vi "Periodic Tasks.vi"(8 "error in":errorcluster) -> ()   [LabVIEW 2017]
doc: "This VI runs in parallel to other tasks. It can contain as many user-defined periodic loops as you need. These can carry out PID or other sorts of timed response."
uses:
  <vilib>/Rock Robotics/WPI/Solenoid/WPI_SolenoidValue.ctl
  <vilib>/Rock Robotics/WPI/ThirdParty/Phoenix-LabVIEW/Motor Controller/Controls/CTRE_Phoenix_MotorControl_ControlMode.ctl
  <vilib>/Rock Robotics/WPI/DriverStation/WPI_DriverStationRobotMode2.ctl
  LabVIEW_is_Under_Control.lib/Util/Toggle/Change Detect.vi
  LabVIEW_is_Under_Control.lib/Util/Toggle/Change Detect Boolean.vi
  Robot Global Data.vi
  <vilib>/Rock Robotics/WPI/Solenoid/WPI_SolenoidSetEnum.vi
panel:
  in  "Exchange":dbl
  in  "ScoringHigh":dbl
  in  "Scoring Low":dbl
  in  "Reset":bool
  in  "Gains Elevador":T1={"proportional gain (Kc)"=1.0, "integral time (Ti, min)"=0.01, "derivative time (Td, min)"=0.0} {"derivative time (Td, min)" format="%.3f"; "integral time (Ti, min)" format="%.3f"; "proportional gain (Kc)" format="%.3f"}
  in  "Range Elevador":cluster{"output high":dbl, "output low":dbl}={"output high"=0.6, "output low"=-0.6} {"output low" format="%.2f"; "output high" format="%.2f"}
  in  "Enable squared":bool
  in  "Score":dbl=-0.3
  in  "Segurando":dbl=0.3
  in  "Expelir":dbl=-0.3
  in  "Coletar":dbl=0.9
  # "Intake"
  # "Drivetrain"
  # "Elevador"
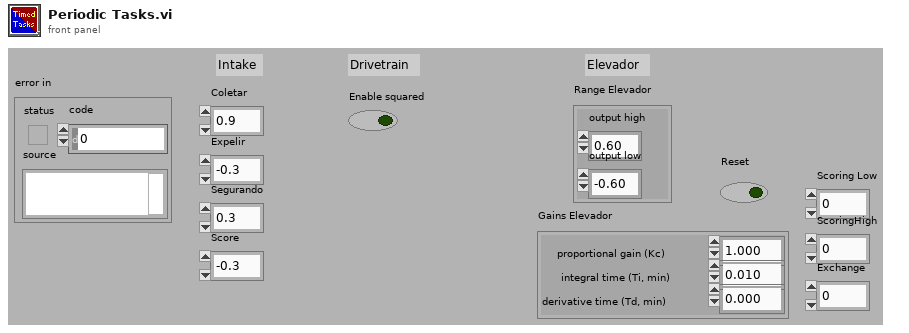
[diagram p1: front panel]
types:
  T1 = cluster{"proportional gain (Kc)":dbl, "integral time (Ti, min)":dbl, "derivative time (Td, min)":dbl}
  T2 = typedef "Máquina de estado do elevador.ctl" = enum16{"Resting", "Scoring Low", "Scoring Higher", "Exchange"}
  T3 = enum16{"Repouso", "Coletando", "Segurando", "Score"}
  T4 = typedef "WPI_SwitchDevRef.ctl" = cluster{"DevStatus":errorcluster, "DIO Channel":T5, "CntIndex":T6, "Normally Closed":bool}
  T5 = typedef "FPGA_DIOChannel.ctl" = enum8{"DIO 0", "DIO 1", "DIO 2", "DIO 3", "DIO 4", "DIO 5", "DIO 6", "DIO 7", "DIO 8", "DIO 9", "DIO MXP 0", "DIO MXP 1", "DIO MXP 2", "DIO MXP 3", "DIO MXP 4", "DIO MXP 5", "DIO MXP 6", "DIO MXP 7", "DIO MXP 8", "DIO MXP 9", "DIO MXP 10", "DIO MXP 11", "DIO MXP 12", "DIO MXP 13", "DIO MXP 14", "DIO MXP 15", "SPI Port CS1", "SPI Port CS2", "SPI Port CS3", "SPI Port MISO", "SPI Port MOSI", "Invalid"}
  T6 = typedef "FPGA_CounterCtrSystemIndex.ctl" = enum8{"Ctr 0", "Ctr 1", "Ctr 2", "Ctr 3", "Ctr 4", "Ctr 5", "Ctr 6", "Ctr 7", "Invalid"}
  T7 = typedef "WPI_EncoderDevRef.ctl" = cluster{"DevStatus":errorcluster, "EncoderIndex":T8, "CounterIndex":T6, "DistancePerCount":dbl, "Decoding Type":T9}
  T8 = typedef "FPGA_EncoderIdx.ctl" = enum8{"Enc 0", "Enc 1", "Enc 2", "Enc 3", "Enc 4", "Enc 5", "Enc 6", "Enc 7", "Invalid"}
  T9 = typedef "WPI_EncoderType.ctl" = enum16{"1x", "2x", "4x"}
  T10 = typedef "WPI_SolenoidDevRef.ctl" = cluster{"DevStatus":errorcluster, "Pneumatics Control Module":u8, "Forward Solenoid Channel":T11, "Reverse Solenoid Channel":T11}
  T11 = typedef "WPI_SolenoidChannel.ctl" = enum8{"Solenoid 0", "Solenoid 1", "Solenoid 2", "Solenoid 3", "Solenoid 4", "Solenoid 5", "Solenoid 6", "Solenoid 7", "Invalid"}
  T12 = typedef "WPI_MotorControlDeviceRef.ctl" = cluster{"DeviceStatus":errorcluster, "Type":T13, "PWM":cluster{"PWM Channel":T14, "DeadBand":T15}, "CAN":cluster{"Device Number":u8, "SetOutput VI Ref":variant, "GetOutput VI Ref":variant, "Enable VI Ref":variant, "Disable VI Ref":variant, "Data":variant}, "Invert":bool, "DIO PWM":cluster{"PWM \"Enable\" Channel":T14, "DIOChannel":T5, "PWM Rate":dbl}}
  T13 = typedef "WPI_MotorControlType.ctl" = enum16{"PWM", "CAN", "DIO PWM"}
  T14 = typedef "FPGA_DIOPWMChannel.ctl" = enum8{"PWM 0", "PWM 1", "PWM 2", "PWM 3", "PWM 4", "PWM 5", "PWM 6", "PWM 7", "PWM 8", "PWM 9", "PWM MXP 0", "PWM MXP 1", "PWM MXP 2", "PWM MXP 3", "PWM MXP 4", "PWM MXP 5", "PWM MXP 6", "PWM MXP 7", "PWM MXP 8", "PWM MXP 9", "Invalid"}
  T15 = typedef "WPI_PWMDeadband.ctl" = cluster{"Name":string, "maxPositivePwm":i32, "minPositivePwm":i32, "centerPwm":i32, "maxNegativePwm":i32, "minNegativePwm":i32, "angularRange":u16}
  T16 = typedef "WPI_SolenoidValue.ctl" = enum16{"Off", "On", "Forward", "Reverse"}
  T17 = typedef "WPI_DriverStationRobotMode2.ctl" = enum16{"Autonomous Disabled", "Autonomous Enabled", "Teleop Disabled", "Teleop Enabled", "Disconnected", "Finish", "Test Disabled", "Test Enabled", "Emergency Stopped"}
  T18 = typedef "CTRE_Phoenix_MotorControl_ControlMode.ctl" = u16
  T19 = typedef "Axes Cluster.ctl" = cluster{"Axes[0]":dbl, "Axes[1]":dbl, "Axes[2]":dbl, "Axes[3]":dbl, "Axes[4]":dbl, "Axes[5]":dbl, "Axes[6]":dbl, "Axes[7]":dbl, "Axes[8]":dbl}
  T20 = typedef "Button Cluster.ctl" = cluster{"Buttons[0]":bool, "Buttons[1]":bool, "Buttons[2]":bool, "Buttons[3]":bool, "Buttons[4]":bool, "Buttons[5]":bool, "Buttons[6]":bool, "Buttons[7]":bool, "Buttons[8]":bool, "Buttons[9]":bool}
  T21 = typedef "D-Pad.ctl" = cluster{"Top":bool, "Bottom":bool, "None":bool, "Right":bool, "Left":bool}
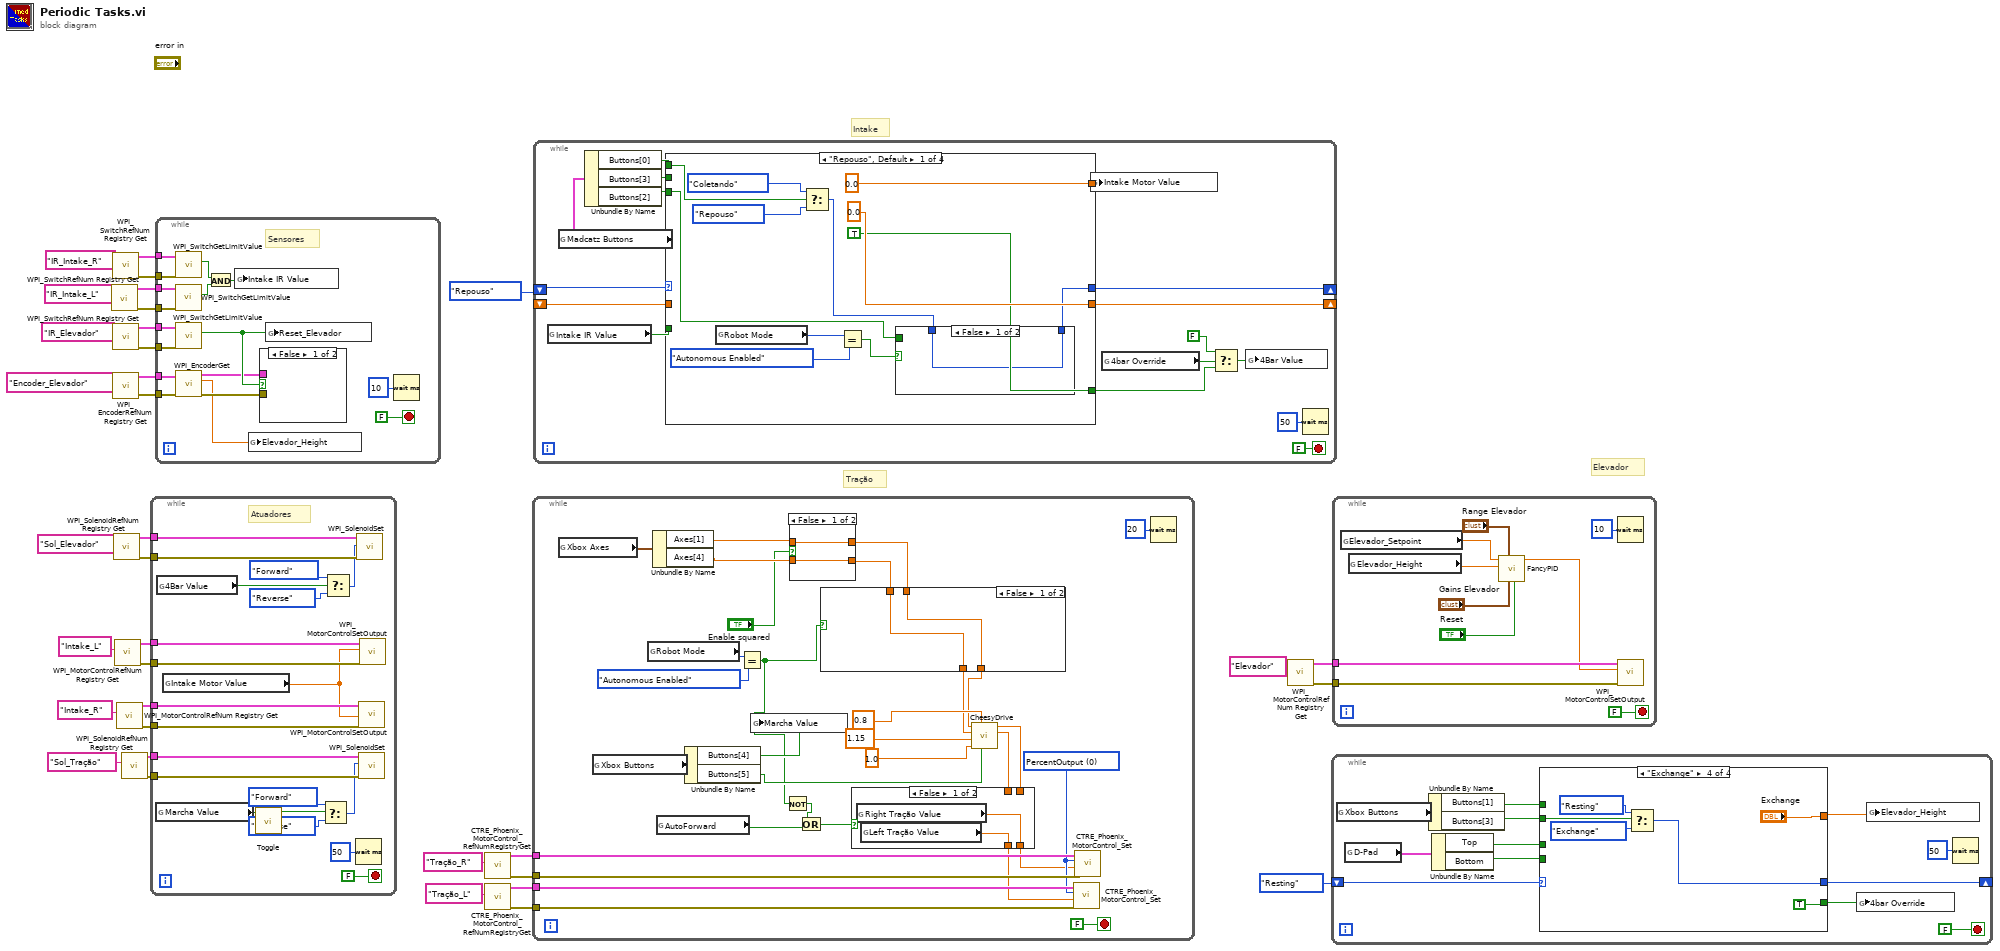
[diagram p0: block diagram]
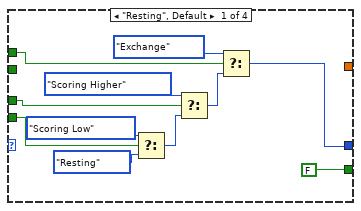
[diagram p2: hidden frame]
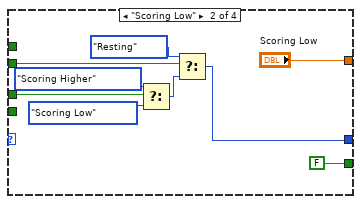
[diagram p3: hidden frame]
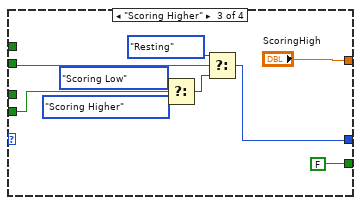
[diagram p4: hidden frame]
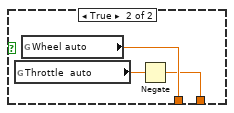
[diagram p6: hidden frame]
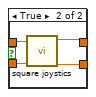
[diagram p7: hidden frame]
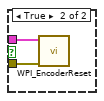
[diagram p8: hidden frame]
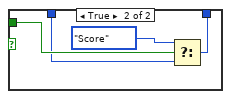
[diagram p9: hidden frame]
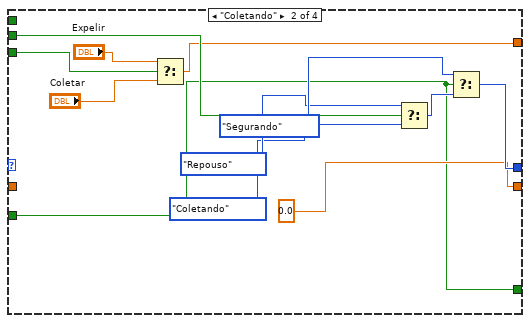
[diagram p10: hidden frame]
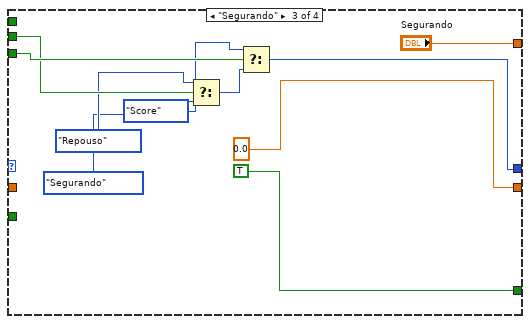
[diagram p11: hidden frame]
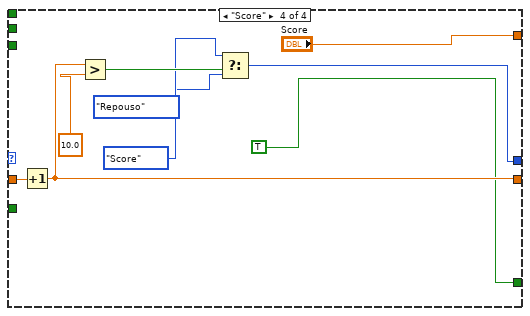
[diagram p12: hidden frame]
diagram:
  # "Elevador"
  # "Tração"
  # "Intake"
  n1 = call <vilib>:"WPI_SwitchRefNum Registry Get.vi"("refnum name"="IR_Intake_L") -> ("error out"=w32:errorcluster, "SwitchDevRef"=w31:T4)  [unwired: 9 in]
  n2 = call <vilib>:"WPI_SwitchRefNum Registry Get.vi"("refnum name"="IR_Intake_R") -> ("error out"=w30:errorcluster, "SwitchDevRef"=w29:T4)  [unwired: 9 in]
  n3 = call <vilib>:"WPI_SwitchRefNum Registry Get.vi"("refnum name"="IR_Elevador") -> ("error out"=w9:errorcluster, "SwitchDevRef"=w10:T4)  [unwired: 9 in]
  n4 = call <vilib>:"WPI_EncoderRefNum Registry Get.vi"("refnum name"="Encoder_Elevador") -> ("error out"=w5:errorcluster, "EncoderDevRef"=w6:T7)  [unwired: 9 in]
  n5 = call <vilib>:"WPI_SolenoidRefNum Registry Get.vi"("refnum name"="Sol_Elevador") -> ("error out"=w27:errorcluster, "SolenoidDevRef"=w26:T10)  [unwired: 9 in]
  n6 = call <vilib>:"WPI_MotorControlRefNum Registry Get.vi"("refnum name"="Intake_L") -> ("error out"=w25:errorcluster, "MotorControlDevRef"=w24:T12)  [unwired: 9 in]
  n7 = call <vilib>:"WPI_MotorControlRefNum Registry Get.vi"("refnum name"="Intake_R") -> ("error out"=w20:errorcluster, "MotorControlDevRef"=w21:T12)  [unwired: 9 in]
  n8 = call <vilib>:"WPI_SolenoidRefNum Registry Get.vi"("refnum name"="Sol_Tração") -> ("error out"=w17:errorcluster, "SolenoidDevRef"=w18:T10)  [unwired: 9 in]
  n9 = while {
    tunnel: w27 -> [w55]
    tunnel: w26 -> [w54]
    tunnel: w25 -> [w49]
    tunnel: w24 -> [w48]
    tunnel: w21 -> [w47]
    tunnel: w20 -> [w46]
    tunnel: w18 -> [w40]
    tunnel: w17 -> [w39]
    stop <- FALSE stop-if-true
    # "Atuadores"
    n10 = global read "Robot Global Data.vi" "Marcha Value"() -> (w37:bool)
    n11 = global read "Robot Global Data.vi" "4Bar Value"() -> (w50:bool)
    n12 = global read "Robot Global Data.vi" "Intake Motor Value"() -> (w45:dbl)
    n13 = call "Toggle.vi"("In"=w37) -> ("Toggled"=w36:bool)  [unwired: 10 in]
    n14 = Select(t=WPI_SolenoidValue."Forward" ("Value"), s=w36, f=WPI_SolenoidValue."Reverse" ("Value")) -> (s? t:f=w38:T16)
    n15 = Select(t=WPI_SolenoidValue."Forward" ("Value"), s=w50, f=WPI_SolenoidValue."Reverse" ("Value")) -> (s? t:f=w53:T16)
    n16 = Wait (ms)(milliseconds to wait=u32 50) -> ()  [unwired: 1 out]
    n17 = call-poly <vilib>:"WPI_SolenoidSet.vi"("error in (no error)"=w55, "Value"=w53, "SolenoidDevRef"=w54) -> ()  [unwired: 7 in, 2 out]
    n18 = call <vilib>:"WPI_MotorControlSetOutput.vi"("error in (no error)"=w46, "Output"=w45, "MotorControlDevRef"=w47) -> ()  [unwired: 6 in, 3 out]
    n19 = call-poly <vilib>:"WPI_SolenoidSet.vi"("error in (no error)"=w39, "Value"=w38, "SolenoidDevRef"=w40) -> ()  [unwired: 7 in, 2 out]
    n20 = call <vilib>:"WPI_MotorControlSetOutput.vi"("error in (no error)"=w49, "Output"=w45, "MotorControlDevRef"=w48) -> ()  [unwired: 6 in, 3 out]
  }
  n21 = while {
    tunnel: w32 -> [w67]
    tunnel: w31 -> [w66]
    tunnel: w30 -> [w65]
    tunnel: w29 -> [w64]
    tunnel: w9 -> [w62]
    tunnel: w10 -> [w63]
    tunnel: w6 -> [w61]
    tunnel: w5 -> [w60]
    stop <- FALSE stop-if-true
    # "Sensores"
    n22 = call <vilib>:"WPI_SwitchGetLimitValue.vi"("error in (no error)"=w67, "SwitchDevRef"=w66) -> ("Switch Pressed"=w72:bool)  [unwired: 7 in, 2 out]
    n23 = call <vilib>:"WPI_SwitchGetLimitValue.vi"("error in (no error)"=w65, "SwitchDevRef"=w64) -> ("Switch Pressed"=w71:bool)  [unwired: 7 in, 2 out]
    n24 = call <vilib>:"WPI_SwitchGetLimitValue.vi"("error in (no error)"=w62, "SwitchDevRef"=w63) -> ("Switch Pressed"=w59:bool)  [unwired: 7 in, 2 out]
    n25 = call <vilib>:"WPI_EncoderGet.vi"("error in (no error)"=w60, "EncoderDevRef"=w61) -> ("error out"=w57:errorcluster, "Distance"=w56:dbl, "EncoderDevRef"=w58:T7)  [unwired: 4 in, 3 out]
    n26 = And(x=w71, y=w72) -> (x .and. y?=w68:bool)
    n27 = global write "Robot Global Data.vi" "Intake IR Value"(w68) -> ()
    n28 = global write "Robot Global Data.vi" "Elevador_Height"(w56) -> ()
    n29 = case shown="False" w59 {
      tunnel: w58 -> [_ w74]
      tunnel: w57 -> [_ w73]
      frame False {
      }
      frame True {
        n30 = call <vilib>:"WPI_EncoderReset.vi"("error in (no error)"=w73, "EncoderDevRef"=w74) -> ()  [unwired: 8 in, 2 out]
      }
    }
    n31 = global write "Robot Global Data.vi" "Reset_Elevador"(w59) -> ()
    n32 = Wait (ms)(milliseconds to wait=u32 10) -> ()  [unwired: 1 out]
  }
  n33 = call <vilib>:"CTRE_Phoenix_MotorControl_RefNumRegistryGet.vi"("refnum name"="Tração_R") -> ("error out"=w12:errorcluster, "PhoenixMotorControlDevRef"=w14:T12)  [unwired: 9 in]
  n34 = call <vilib>:"CTRE_Phoenix_MotorControl_RefNumRegistryGet.vi"("refnum name"="Tração_L") -> ("error out"=w11:errorcluster, "PhoenixMotorControlDevRef"=w13:T12)  [unwired: 9 in]
  n35 = while {
    tunnel: w14 -> [w96]
    tunnel: w13 -> [w95]
    tunnel: w12 -> [w94]
    tunnel: w11 -> [w93]
    stop <- FALSE stop-if-true
    w92 = T18 0 items=["PercentOutput"=0, "Position"=1, "Velocity"=2, "Current"=3, "Follower"=5, "MotionProfile"=6, "MotionMagic"=7, "MotionMagicArc"=8, "MotionProfileArc"=10, "Disabled"=15] ("Control Mode")
    n36 = global read "Robot Global Data.vi" "Xbox Axes"() -> (w105:T19)
    n37 = global read "Robot Global Data.vi" "Xbox Buttons"() -> (w103:T20)
    n38 = global read "Robot Global Data.vi" "Robot Mode"() -> (w88:T17)
    n39 = Unbundle By Name(w105) -> ("Axes[1]"=w90:dbl, "Axes[4]"=w91:dbl)
    n40 = global read "Robot Global Data.vi" "AutoForward"() -> (w76:bool)
    n41 = Unbundle By Name(w103) -> ("Buttons[4]"=w101:bool, "Buttons[5]"=w102:bool)
    n42 = Equal?(x=w88, y=WPI_DriverStationRobotMode2."Autonomous Enabled") -> (x = y?=w75:bool)
    n43 = global write "Robot Global Data.vi" "Marcha Value"(w101) -> ()
    n44 = Not(x=w75) -> (.not. x?=w78:bool)
    n45 = case shown="False" "Enable squared" {
      tunnel: w91 -> [w116 w120]
      tunnel: [w116 w119] -> w85
      tunnel: w90 -> [w115 w118]
      tunnel: [w115 w117] -> w86
      frame False {
      }
      frame True {
        n46 = call "square joystics.vi"("right joy"=w120, "left joy"=w118) -> ("Right Out"=w119:dbl, "Left Out"=w117:dbl)  [unwired: 8 in]
      }
    }
    n47 = Or(x=w78, y=w76) -> (x .or. y?=w77:bool)
    n48 = case shown="False" w75 {
      tunnel: [w110 w114] -> w79
      tunnel: [w111 w112] -> w80
      tunnel: w86 -> [w111 _]
      tunnel: w85 -> [w110 _]
      frame False {
      }
      frame True {
        n49 = global read "Robot Global Data.vi" "Throttle  auto"() -> (w113:dbl)
        n50 = global read "Robot Global Data.vi" "Wheel auto"() -> (w114:dbl)
        n51 = Negate(x=w113) -> (-x=w112:dbl)
      }
    }
    n52 = call "CheesyDrive.vi"("Quickturn"=w102, "WheelNonLinearity"=0.8, "negInertiaScalar"=1.0, "Sensitivty"=1.15, "Wheel"=w79, "Throttle"=w80) -> ("Right PWM"=w81:dbl, "Left PWM"=w83:dbl)  [unwired: 4 in]
    n53 = case shown="False" w77 {
      tunnel: [w106 w108] -> w84
      tunnel: w83 -> [_ w108]
      tunnel: [w107 w109] -> w82
      tunnel: w81 -> [_ w109]
      frame False {
        n54 = global read "Robot Global Data.vi" "Right Tração Value"() -> (w106:dbl)
        n55 = global read "Robot Global Data.vi" "Left Tração Value"() -> (w107:dbl)
      }
      frame True {
      }
    }
    n56 = call <vilib>:"CTRE_Phoenix_MotorControl_Set.vi"("error in (no error)"=w93, "Output"=w82, "Control Mode"=w92, "PhoenixMotorControlDevRef"=w95) -> ()  [unwired: 6 in, 2 out]
    n57 = call <vilib>:"CTRE_Phoenix_MotorControl_Set.vi"("error in (no error)"=w94, "Output"=w84, "Control Mode"=w92, "PhoenixMotorControlDevRef"=w96) -> ()  [unwired: 6 in, 2 out]
    n58 = Wait (ms)(milliseconds to wait=u32 20) -> ()  [unwired: 1 out]
  }
  n59 = while {
    shift-right: [w132] -> _
    shift-left: T3."Repouso" -> [w136]
    shift-right: [w129] -> _
    shift-left: _ -> [w130]
    stop <- FALSE stop-if-true
    n60 = global read "Robot Global Data.vi" "Intake IR Value"() -> (w131:bool)
    n61 = global read "Robot Global Data.vi" "Madcatz Buttons"() -> (w133:T20)
    n62 = Unbundle By Name(w133) -> ("Buttons[0]"=w125:bool, "Buttons[3]"=w127:bool, "Buttons[2]"=w126:bool)
    n63 = case shown="\"Repouso\", Default" w136 {
      tunnel: w125 -> [w148 _ _ _]
      tunnel: [w138 w161 w169 w178] -> w132
      tunnel: w127 -> [_ w164 w173 _]
      tunnel: w131 -> [_ w155 _ _]
      tunnel: w126 -> [w137 w154 w175 _]
      tunnel: w130 -> [_ _ _ w184]
      tunnel: [0.0 0.0 0.0 w183] -> w129
      tunnel: [0.0 w156 "Segurando" "Score"] -> w128
      tunnel: [TRUE w155 TRUE TRUE] -> w123
      frame "Repouso", Default {
        n64 = global read "Robot Global Data.vi" "Robot Mode"() -> (w141:T17)
        n65 = Select(t=T3."Coletando", s=w148, f=T3."Repouso") -> (s? t:f=w139:T3)
        n66 = Equal?(x=w141, y=WPI_DriverStationRobotMode2."Autonomous Enabled") -> (x = y?=w140:bool)
        n67 = case shown="False" w140 {
          tunnel: w137 -> [_ w153]
          tunnel: w139 -> [w149 w152]
          tunnel: [w149 w150] -> w138
          frame False {
          }
          frame True {
            n68 = Select(t=T3."Score", s=w153, f=w152) -> (s? t:f=w150:T3)
          }
        }
      }
      frame "Coletando" {
        n69 = Select(t="Expelir", s=w154, f="Coletar") -> (s? t:f=w156:dbl)
        n70 = Select(t=T3."Repouso", s=w164, f=T3."Coletando") -> (s? t:f=w158:T3)
        n71 = Select(t=T3."Segurando", s=w155, f=w158) -> (s? t:f=w161:T3)
      }
      frame "Segurando" {
        n72 = Select(t=T3."Repouso", s=w173, f=T3."Segurando") -> (s? t:f=w172:T3)
        n73 = Select(t=T3."Score", s=w175, f=w172) -> (s? t:f=w169:T3)
      }
      frame "Score" {
        n74 = Increment(x=w184) -> (x+1=w183:dbl)
        n75 = Greater?(x=w183, y=10.0) -> (0:w181:bool)
        n76 = Select(t=T3."Repouso", s=w181, f=T3."Score") -> (s? t:f=w178:T3)
      }
    }
    n77 = global write "Robot Global Data.vi" "Intake Motor Value"(w128) -> ()
    n78 = global read "Robot Global Data.vi" "4bar Override"() -> (w124:bool)
    n79 = Select(t=FALSE, s=w124, f=w123) -> (s? t:f=w121:bool)
    n80 = global write "Robot Global Data.vi" "4Bar Value"(w121) -> ()
    n81 = Wait (ms)(milliseconds to wait=u32 50) -> ()  [unwired: 1 out]
  }
  n82 = call <vilib>:"WPI_MotorControlRefNum Registry Get.vi"("refnum name"="Elevador") -> ("error out"=w2:errorcluster, "MotorControlDevRef"=w3:T12)  [unwired: 9 in]
  n83 = while {
    shift-right: [w186] -> _
    shift-left: Máquina_de_estado_do_elevador."Resting" -> [w187]
    stop <- FALSE stop-if-true
    n84 = global read "Robot Global Data.vi" "Xbox Buttons"() -> (w193:T20)
    n85 = global read "Robot Global Data.vi" "D-Pad"() -> (w194:T21)
    n86 = Unbundle By Name(w193) -> ("Buttons[1]"=w188:bool, "Buttons[3]"=w192:bool)
    n87 = Unbundle By Name(w194) -> ("Top"=w191:bool, "Bottom"=w190:bool)
    n88 = case shown="\"Exchange\"" w187 {
      tunnel: w192 -> [_ w215 w224 w230]
      tunnel: w191 -> [w206 w214 _ _]
      tunnel: w190 -> [w205 _ w222 _]
      tunnel: [_ "Scoring Low" "ScoringHigh" "Exchange"] -> w189
      tunnel: [w198 w212 w221 w229] -> w186
      tunnel: w188 -> [w203 _ _ _]
      tunnel: [FALSE FALSE FALSE TRUE] -> w185
      frame "Resting", Default {
        n89 = Select(t=Máquina_de_estado_do_elevador."Scoring Low", s=w205, f=Máquina_de_estado_do_elevador."Resting") -> (s? t:f=w207:T2)
        n90 = Select(t=Máquina_de_estado_do_elevador."Scoring Higher", s=w206, f=w207) -> (s? t:f=w204:T2)
        n91 = Select(t=Máquina_de_estado_do_elevador."Exchange", s=w203, f=w204) -> (s? t:f=w198:T2)
      }
      frame "Scoring Low" {
        n92 = Select(t=Máquina_de_estado_do_elevador."Scoring Higher", s=w214, f=Máquina_de_estado_do_elevador."Scoring Low") -> (s? t:f=w213:T2)
        n93 = Select(t=Máquina_de_estado_do_elevador."Resting", s=w215, f=w213) -> (s? t:f=w212:T2)
      }
      frame "Scoring Higher" {
        n94 = Select(t=Máquina_de_estado_do_elevador."Scoring Low", s=w222, f=Máquina_de_estado_do_elevador."Scoring Higher") -> (s? t:f=w223:T2)
        n95 = Select(t=Máquina_de_estado_do_elevador."Resting", s=w224, f=w223) -> (s? t:f=w221:T2)
      }
      frame "Exchange" {
        n96 = Select(t=Máquina_de_estado_do_elevador."Resting", s=w230, f=Máquina_de_estado_do_elevador."Exchange") -> (s? t:f=w229:T2)
      }
    }
    n97 = global write "Robot Global Data.vi" "4bar Override"(w185) -> ()
    n98 = global write "Robot Global Data.vi" "Elevador_Height"(w189) -> ()
    n99 = Wait (ms)(milliseconds to wait=u32 50) -> ()  [unwired: 1 out]
  }
  n100 = while {
    tunnel: w3 -> [w239]
    tunnel: w2 -> [w238]
    stop <- FALSE stop-if-true
    n101 = global read "Robot Global Data.vi" "Elevador_Setpoint"() -> (w233:dbl)
    n102 = global read "Robot Global Data.vi" "Elevador_Height"() -> (w232:dbl)
    n103 = call "FancyPID.vi"("Reset"="Reset", "Gains"="Gains Elevador", "Range"="Range Elevador", "Process variable"=w232, "Setpoint"=w233) -> ("output"=w237:dbl)  [unwired: 6 in]
    n104 = Wait (ms)(milliseconds to wait=u32 10) -> ()  [unwired: 1 out]
    n105 = call <vilib>:"WPI_MotorControlSetOutput.vi"("error in (no error)"=w238, "Output"=w237, "MotorControlDevRef"=w239) -> ()  [unwired: 6 in, 3 out]
  }
